vi "Heartbeat State Manager.vi"(8 "Error In":errorcluster, 9 "Heartbeat state manager Input VI names":T6, 11 "HB Command Event IN":refnum<user-event>) -> (0 "Error Out":errorcluster, 1 "Error conditions Cluster":T4, 2 "Master-Slave messaging Flags":T5={"Instruction available"=TRUE, "Slave action completed"=TRUE, "Slave Ready?"=FALSE}, 3 "Heartbeat information cluster":T1, 4 "Slave Completions Received":i32, 5 "Master Instructions Issued":i32)   [LabVIEW 2012]
doc: "SciScan 1.2 160622\nThis VI MUST be used in all VIs which make use of heartbeats for synchronisation with a client or slave"
uses:
  Heartbeat state manager Input VI names.ctl
  Master Slave messaging Flags.ctl
  Custom Controls and Typedefs/HB_Error Conditions Cluster.ctl
  Custom Controls and Typedefs/Heartbeat information cluster.ctl
  Custom Controls and Typedefs/Heartbeat Event Source.ctl
  Custom Controls/Heartbeat_States.ctl
  Custom Controls and Typedefs/HB Actionable Event.ctl
  Broken Chain FGV Command.ctl
  CommonResource VIs/Timing/Timer Commands.ctl
  Custom Controls and Typedefs/HFG Commands.ctl
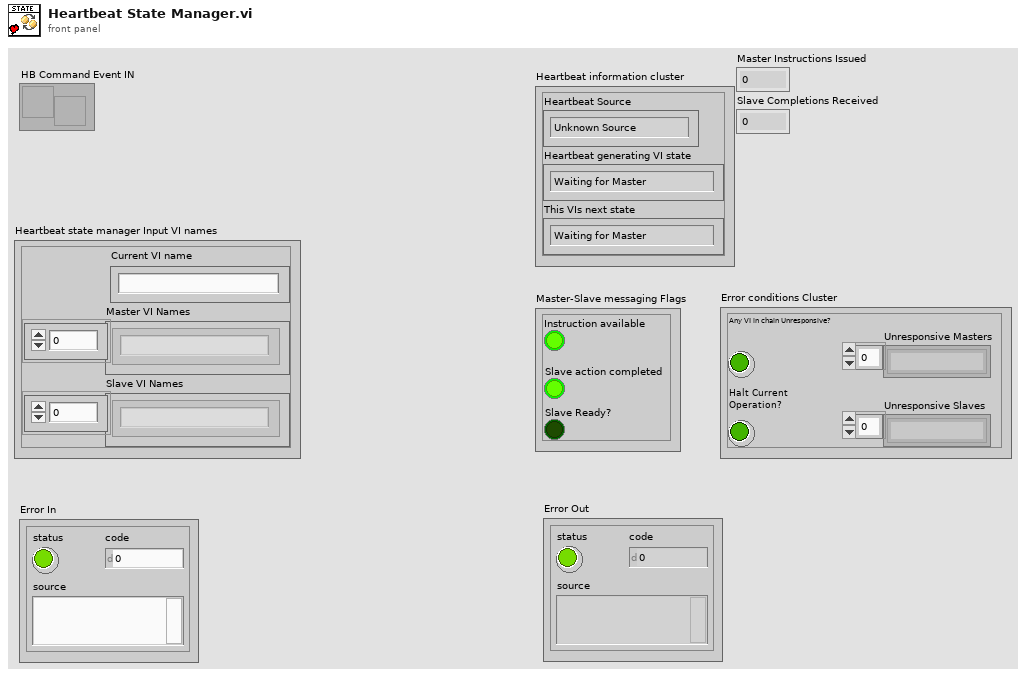
[diagram p1: front panel]
types:
  T1 = typedef "Heartbeat information cluster.ctl" = cluster{"Heartbeat Source":T2, "Heartbeat generating VI state":T3, "This VIs next state":T3}
  T2 = typedef "Heartbeat Event Source.ctl" = enum16{"Unknown Source", "Timeout", "This VI", "Master", "Slave"}
  T3 = typedef "Heartbeat_States.ctl" = enum16{"Waiting for Master", "Instruction Issued", "Waiting for Slave Completion", "Completed", "Cancelled", "Failed", "Broken Link"}
  T4 = typedef "HB_Error Conditions Cluster.ctl" = cluster{"Any VI in chain Unresponsive?":bool, "Halt Current Operation?":bool, "Unresponsive Masters":string[], "Unresponsive Slaves":string[]}
  T5 = typedef "Master Slave messaging Flags.ctl" = cluster{"Instruction available":bool, "Slave action completed":bool, "Slave Ready?":bool}
  T6 = typedef "Heartbeat state manager Input VI names.ctl" = cluster{"Current VI name":string, "Master VI Names":string[], "Slave VI Names":string[]}
  T7 = typedef "Broken Chain FGV Command.ctl" = enum16{"Initialize", "Update VI status", "Get All VI status"}
  T8 = cluster{"Master VI Names":string[], "Slave VI Names":string[]}
  T9 = typedef "HFG Commands.ctl" = enum16{"Set", "Get", "Initialize"}
  T10 = typedef "Timer Commands.ctl" = enum16{"Clear All", "Start", "Pause", "Check Time"}
  T11 = typedef "HB Actionable Event.ctl" = enum16{"Master instruction event", "Slave ready event", "Slave unavailable event", "Cancelled or Failed event", "Slave action complete event", "QUIT", "Broken Link", "Recovered from Broken Link"}
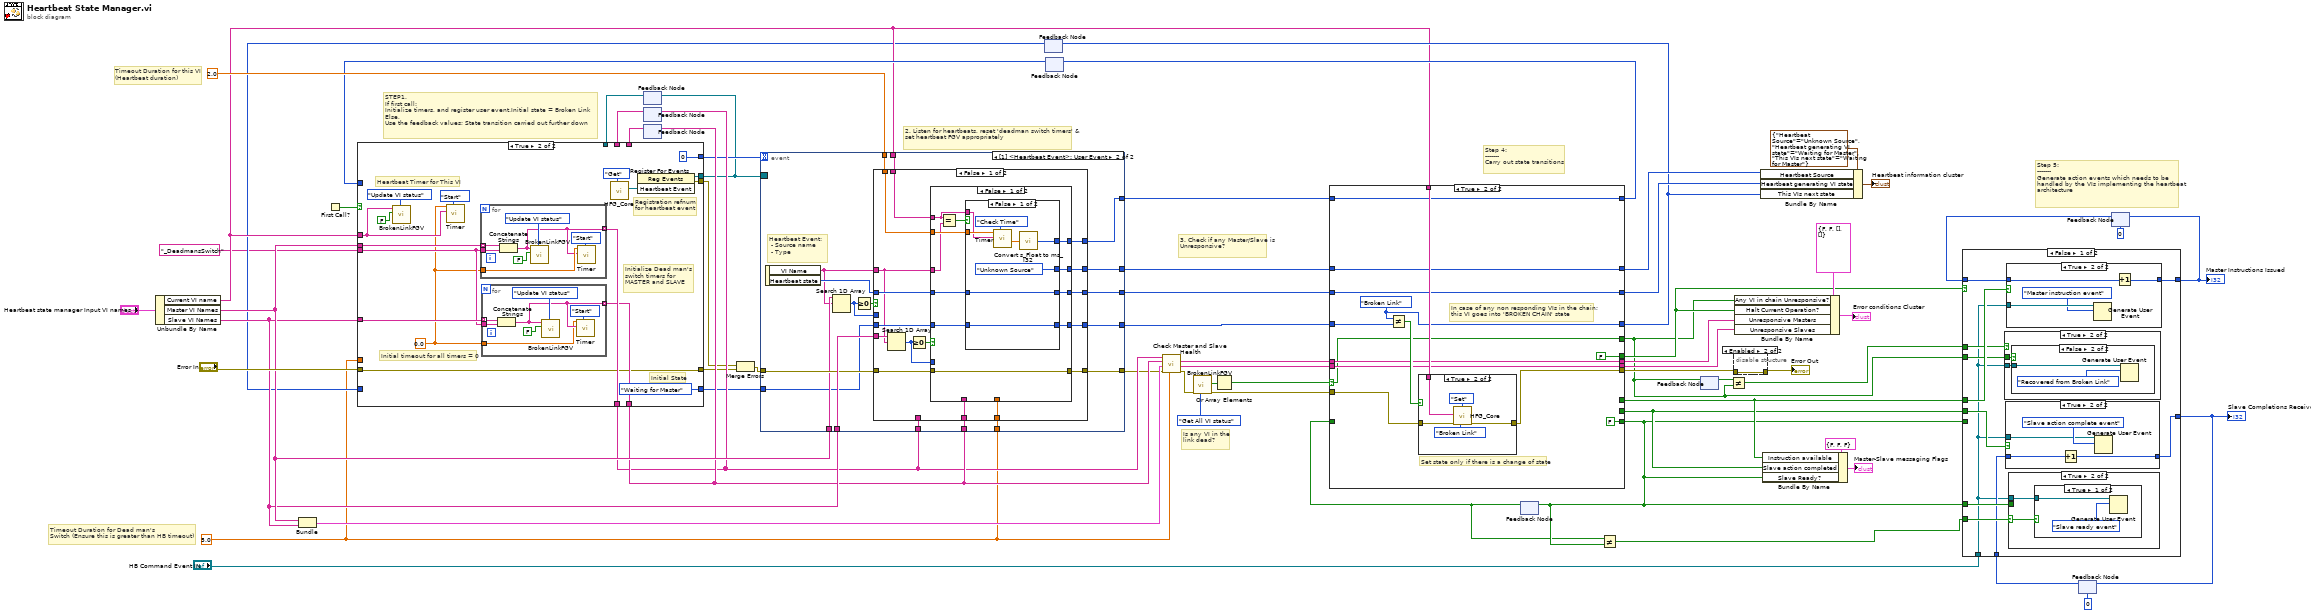
[diagram p0: block diagram]
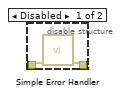
[diagram p2: hidden frame]
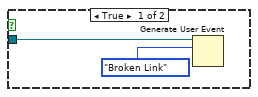
[diagram p4: hidden frame]
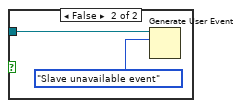
[diagram p7: hidden frame]
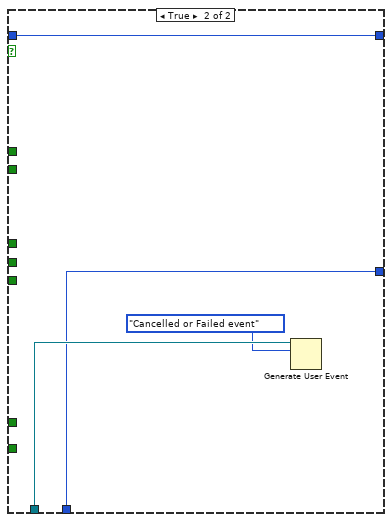
[diagram p9: hidden frame]
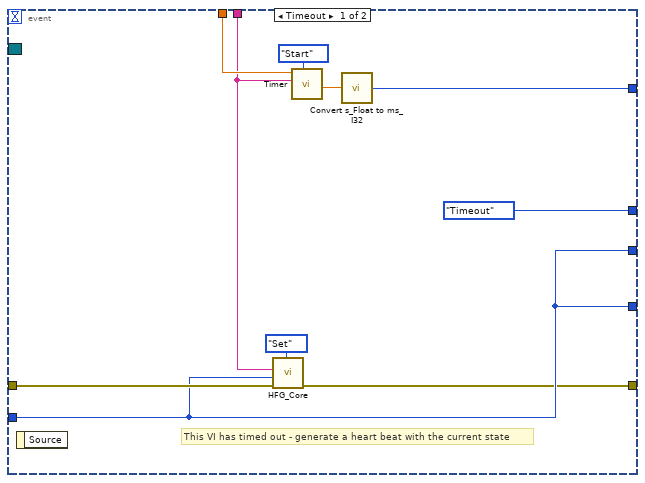
[diagram p10: hidden frame]
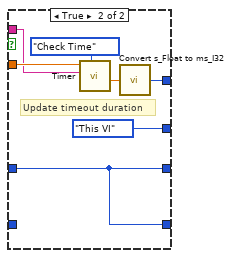
[diagram p11: hidden frame]
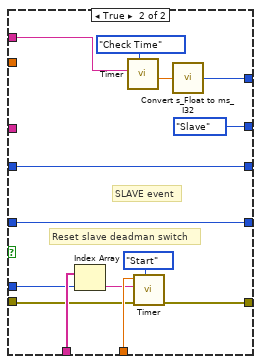
[diagram p12: hidden frame]
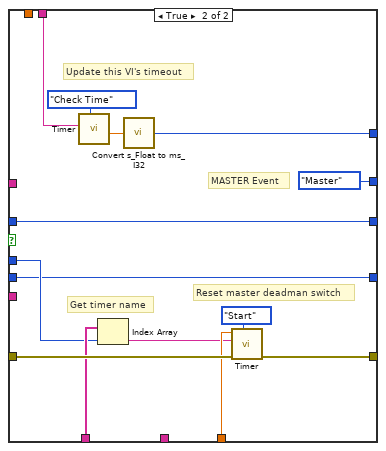
[diagram p13: hidden frame]
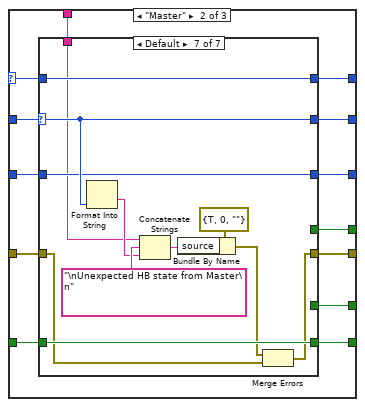
[diagram p16: hidden frame]
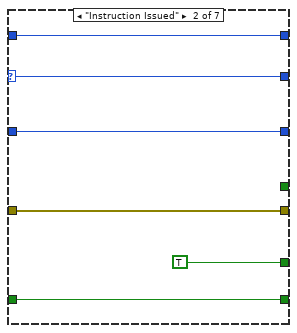
[diagram p18: hidden frame]
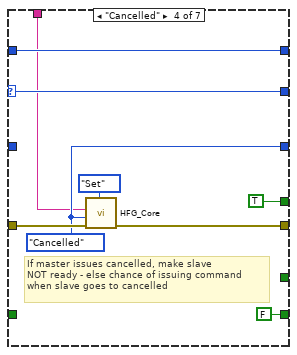
[diagram p20: hidden frame]
diagram:
  w27 = 5.0 ("Response time for Master/Slave")
  # "Timeout Duration for Dead man's\nSwitch (Ensure this is greater than HB timeout)"
  # "Step 5:\n-------\nGenerate action events which needs to be handled by the VIs implementing the heartbeat architecture"
  # "Is any VI in the link dead?"
  # "2. Listen for heartbeats, reset 'deadman switch timers' & set heartbeat FGV appropriately"
  # "Timeout Duration for this VI\n(Heartbeat duration)"
  # "Step 4:\n-------\nCarry out state transitions"
  # "3. Check if any Master/Slave is Unresponsive?"
  # "STEP1. \nIf first call:\nInitialize timers, and register user event.Initial state = Broken Link\nElse,\nUse the feedback values; State transition carried out further down"
  n1 = Unbundle By Name("Heartbeat state manager Input VI names") -> ("Current VI name"=w46:string, "Master VI Names"=w45:string[], "Slave VI Names"=w44:string[])
  n2 = Bundle("Master VI Names"=w45, "Slave VI Names"=w44) -> (w60:T8)  [unwired: 1 in]
  n3 = First Call?() -> (First Call?: T/F=w64:bool)
  n4 = feedback #1() -> (w33:refnum<event-registration>)  [unwired: 1 in]
  n5 = feedback #2() -> (w63:string[])  [unwired: 1 in]
  n6 = feedback #3() -> (w62:string[])  [unwired: 1 in]
  n7 = feedback #4() -> (w37:T3)  [unwired: 1 in]
  n8 = feedback #5() -> (w47:i32)  [unwired: 1 in]
  n9 = case shown="True" w64 {
    tunnel: w46 -> [_ w80]
    tunnel: w45 -> [_ w88]
    tunnel: w44 -> [_ w87]
    tunnel: [w71 w86] -> w42
    tunnel: [w70 w85] -> w43
    tunnel: w63 -> [w71 _]
    tunnel: w62 -> [w70 _]
    tunnel: [w69 w84] -> w2
    tunnel: "Error In" -> [w69 w84]
    tunnel: w27 -> [_ _]
    tunnel: [w68 0] -> w35
    tunnel: w47 -> [w68 _]
    tunnel: w37 -> [w67 _]
    tunnel: [w67 Heartbeat_States."Waiting for Master" ("x")] -> w36
    tunnel: [w66 w75] -> w34
    tunnel: w33 -> [w66 _]
    tunnel: "_DeadmansSwitch" ("Current VI name") -> [_ w74]
    tunnel: [_ w72] -> w1
    frame False {
    }
    frame True {
      w73 = 0.0 ("Response time for Master/Slave")
      # "Registration refnum\nfor heartbeat event"
      # "Initial State"
      # "Initialize Dead man's switch timers for MASTER and SLAVE"
      # "Heartbeat Timer for This VI"
      # "Initial timeout for all timers = 0"
      n10 = call "BrokenLinkFGV.vi"("Broken Chain FGV Action"=Broken_Chain_FGV_Command."Update VI status", "Broken?"=FALSE, "String"=w80) -> ()  [unwired: 6 in, 3 out]
      n11 = call "Timer.vi"("Timer Command"=Timer_Commands."Start", "VI name (Optional)"=w80, "Set Time IN (s)"=w73) -> ()  [unwired: 3 in, 6 out]
      n12 = for {
        tunnel: w88 -> [w100] mode=indexing
        tunnel: [w96] -> w86 mode=indexing
        tunnel: w74 -> [w99]
        tunnel: w73 -> [w97]
        n13 = Concatenate Strings(w100, w99) -> (w96:string)
        n14 = call "BrokenLinkFGV.vi"("Broken Chain FGV Action"=Broken_Chain_FGV_Command."Update VI status", "Broken?"=FALSE, "String"=w96) -> ()  [unwired: 6 in, 3 out]
        n15 = call "Timer.vi"("Timer Command"=Timer_Commands."Start", "VI name (Optional)"=w96, "Set Time IN (s)"=w97) -> ()  [unwired: 3 in, 6 out]
      }
      n16 = for {
        tunnel: w87 -> [w93] mode=indexing
        tunnel: [w90] -> w85 mode=indexing
        tunnel: w74 -> [w92]
        tunnel: w73 -> [w89]
        n17 = Concatenate Strings(w93, w92) -> (w90:string)
        n18 = call "BrokenLinkFGV.vi"("Broken Chain FGV Action"=Broken_Chain_FGV_Command."Update VI status", "Broken?"=FALSE, "String"=w90) -> ()  [unwired: 6 in, 3 out]
        n19 = call "Timer.vi"("Timer Command"=Timer_Commands."Start", "VI name (Optional)"=w90, "Set Time IN (s)"=w89) -> ()  [unwired: 3 in, 6 out]
      }
      n20 = call "HFG_Core.vi"("HFG Commands"=HFG_Commands."Get") -> ("Heartbeat Event"=w77:refnum<user-event>)  [unwired: 7 in, 3 out]
      n21 = register-events(w77) -> (reference out=w75:refnum<event-registration>, error out=w72:errorcluster)  [unwired: 2 in]
    }
  }
  n22 = feedback-in #1(w34) -> ()
  n23 = feedback-in #2(w42) -> ()
  n24 = feedback-in #3(w43) -> ()
  n25 = Merge Errors(w1, w2) -> (w3:errorcluster)
  n26 = event shown="[1] <Heartbeat Event>: User Event" {
    selector: w34 -> [_ _]
    dyn-events: _ -> [_ _]
    timeout: w35 -> [_ _]
    tunnel: w36 -> [w105 w120]
    tunnel: [w105 w114] -> w24
    tunnel: 2.0 ("Response time for Master/Slave") -> [w111 w129]
    tunnel: [w106 w128] -> w38
    tunnel: [w105 w117] -> w40
    tunnel: w46 -> [w103 w130]
    tunnel: w3 -> [w109 w123]
    tunnel: [w104 w115] -> w41
    tunnel: [Heartbeat_Event_Source."Timeout" ("Heartbeat Event Types") w127] -> w39
    tunnel: w45 -> [_ w122]
    tunnel: w44 -> [_ w126]
    tunnel: w43 -> [_ w125]
    tunnel: w27 -> [_ w124]
    tunnel: w42 -> [_ w116]
    event Timeout {
      # "This VI has timed out - generate a heart beat with the current state"
      n27 = event-data() -> ()  [unwired: 1 in, 1 out]
      n28 = call "HFG_Core.vi"("HFG Commands"=HFG_Commands."Set", "Error In"=w109, "Heartbeat state IN"=w105, "VI Name (Calling VIs name by default)"=w103) -> ("Error Out"=w104:errorcluster)  [unwired: 4 in, 3 out]
      n29 = call "Timer.vi"("Timer Command"=Timer_Commands."Start", "VI name (Optional)"=w103, "Set Time IN (s)"=w111) -> ("Remaining Time (s)"=w107:dbl)  [unwired: 3 in, 5 out]
      n30 = call "Convert s_Float to ms_I32.vi"("Seconds IN (Float)"=w107) -> ("milliseconds OUT (I32)"=w106:i32)
    }
    event User Event {
      # "Heartbeat Event: \n - Source name\n - Type"
      n31 = event-data() -> ("VI Name"=w113:string, "Heartbeat state"=w118:T3)  [unwired: 1 in]
      n32 = Search 1D Array(1D array=w122, element=w113) -> (index of element=w119:i32)  [unwired: 1 in]
      n33 = Greater Or Equal To 0?(x=w119) -> (x >= 0?=w121:bool)
      n34 = case shown="False" w121 {
        tunnel: w130 -> [w146 w198]
        tunnel: w129 -> [w145 _]
        tunnel: [w144 w197] -> w128
        tunnel: [w143 Heartbeat_Event_Source."Master" ("Heartbeat Event Types")] -> w127
        tunnel: w113 -> [w131 _]
        tunnel: w126 -> [w142 _]
        tunnel: w125 -> [w140 _]
        tunnel: w124 -> [w139 w191]
        tunnel: w123 -> [w137 w194]
        tunnel: w120 -> [w134 w189]
        tunnel: w119 -> [_ w192]
        tunnel: w118 -> [w136 w195]
        tunnel: [w135 w195] -> w117
        tunnel: w116 -> [_ w193]
        tunnel: [w133 w190] -> w115
        tunnel: [w132 w189] -> w114
        frame False {
          n35 = Search 1D Array(1D array=w142, element=w131) -> (index of element=w138:i32)  [unwired: 1 in]
          n36 = Greater Or Equal To 0?(x=w138) -> (x >= 0?=w141:bool)
          n37 = case shown="False" w141 {
            tunnel: w146 -> [w147 w178]
            tunnel: w145 -> [w156 _]
            tunnel: [w155 w180] -> w144
            tunnel: [w154 Heartbeat_Event_Source."Slave" ("Heartbeat Event Types")] -> w143
            tunnel: w131 -> [w153 _]
            tunnel: w140 -> [_ w185]
            tunnel: w139 -> [_ w184]
            tunnel: w138 -> [_ w183]
            tunnel: w137 -> [w152 w179]
            tunnel: w136 -> [w151 w176]
            tunnel: [w149 w176] -> w135
            tunnel: w134 -> [w148 w175]
            tunnel: [w152 w177] -> w133
            tunnel: [w150 w175] -> w132
            frame False {
              n38 = Equal?(x=w147, y=w153) -> (x = y?=w157:bool)
              n39 = case shown="False" w157 {
                tunnel: w156 -> [w164 w171]
                tunnel: [w162 w169] -> w155
                tunnel: [Heartbeat_Event_Source."Unknown Source" ("Heartbeat Event Types") Heartbeat_Event_Source."This VI" ("Heartbeat Event Types")] -> w154
                tunnel: w151 -> [w160 w167]
                tunnel: [w159 w167] -> w150
                tunnel: [w160 w167] -> w149
                tunnel: w148 -> [w159 _]
                tunnel: w147 -> [w158 w166]
                frame False {
                  n40 = call "Timer.vi"("Timer Command"=Timer_Commands."Check Time", "VI name (Optional)"=w158, "Set Time IN (s)"=w164) -> ("Remaining Time (s)"=w163:dbl)  [unwired: 3 in, 5 out]
                  n41 = call "Convert s_Float to ms_I32.vi"("Seconds IN (Float)"=w163) -> ("milliseconds OUT (I32)"=w162:i32)
                }
                frame True {
                  # "Update timeout duration"
                  n42 = call "Timer.vi"("Timer Command"=Timer_Commands."Check Time", "VI name (Optional)"=w166, "Set Time IN (s)"=w171) -> ("Remaining Time (s)"=w170:dbl)  [unwired: 3 in, 5 out]
                  n43 = call "Convert s_Float to ms_I32.vi"("Seconds IN (Float)"=w170) -> ("milliseconds OUT (I32)"=w169:i32)
                }
              }
            }
            frame True {
              # "Reset slave deadman switch"
              # "SLAVE event"
              n44 = Index Array(array=w185, index=w183) -> (element=w173:string)
              n45 = call "Timer.vi"("Timer Command"=Timer_Commands."Check Time", "VI name (Optional)"=w178) -> ("Remaining Time (s)"=w181:dbl)  [unwired: 4 in, 5 out]
              n46 = call "Timer.vi"("Timer Command"=Timer_Commands."Start", "Error In"=w179, "VI name (Optional)"=w173, "Set Time IN (s)"=w184) -> ("Error Out"=w177:errorcluster)  [unwired: 2 in, 5 out]
              n47 = call "Convert s_Float to ms_I32.vi"("Seconds IN (Float)"=w181) -> ("milliseconds OUT (I32)"=w180:i32)
            }
          }
        }
        frame True {
          # "Get timer name"
          # "Update this VI's timeout"
          # "Reset master deadman switch"
          # "MASTER Event"
          n48 = call "Timer.vi"("Timer Command"=Timer_Commands."Check Time", "VI name (Optional)"=w198) -> ("Remaining Time (s)"=w199:dbl)  [unwired: 4 in, 5 out]
          n49 = Index Array(array=w193, index=w192) -> (element=w187:string)
          n50 = call "Convert s_Float to ms_I32.vi"("Seconds IN (Float)"=w199) -> ("milliseconds OUT (I32)"=w197:i32)
          n51 = call "Timer.vi"("Timer Command"=Timer_Commands."Start", "Error In"=w194, "VI name (Optional)"=w187, "Set Time IN (s)"=w191) -> ("Error Out"=w190:errorcluster)  [unwired: 2 in, 5 out]
        }
      }
    }
  }
  n52 = call "Check Master and Slave Health.vi"("Timeout duration"=w27, "Error In"=w41, "Master and Slave VI names"=w60, "Slave timer names array"=w43, "Master timer names array"=w42) -> ("Error Out"=w30:errorcluster, "Unresponsive Slaves"=w7:string[], "Unresponsive Masters"=w8:string[])  [unwired: 3 in, 1 out]
  n53 = call "BrokenLinkFGV.vi"("Broken Chain FGV Action"=Broken_Chain_FGV_Command."Get All VI status", "Error In"=w30) -> ("Error Out"=w28:errorcluster, "VI broken? array"=w32:bool[])  [unwired: 7 in, 1 out]
  n54 = Or Array Elements(Boolean array=w32) -> (logical OR=w29:bool)
  n55 = feedback #6() -> (w13:bool)  [unwired: 1 in]
  n56 = case shown="True" w29 {
    selector: w29 -> [_ w528]
    tunnel: w28 -> [w213 w539]
    tunnel: w24 -> [w215 w541]
    tunnel: w40 -> [w210 w536]
    tunnel: w39 -> [w208 w535]
    tunnel: [w202 FALSE ("Halt Current Operation")] -> w16
    tunnel: w46 -> [w212 w538]
    tunnel: [w214 w537] -> w50
    tunnel: [w209 w536] -> w52
    tunnel: [w207 w535] -> w51
    tunnel: [_ w528] -> w4
    tunnel: w8 -> [_ w534]
    tunnel: w7 -> [_ w533]
    tunnel: [_ w534] -> w55
    tunnel: [_ w533] -> w54
    tunnel: [w211 w531] -> w26
    tunnel: [w206 _] -> w21
    tunnel: [w205 _] -> w15
    tunnel: [w204 FALSE] -> w14
    tunnel: w13 -> [w203 _]
    tunnel: w38 -> [w201 w529]
    tunnel: [w201 w529] -> w48
    frame False {
      n57 = case shown="\"Waiting for Master\"" w215 {
        selector: w215 -> [w224 _ w397 _ _]
        tunnel: [w225 w350 w398 w515 w526] -> w214
        tunnel: w213 -> [w220 w345 w393 w517 w521]
        tunnel: w212 -> [w219 w351 w392 w516 w527]
        tunnel: [w221 w344 w394 w514 w525] -> w211
        tunnel: [w223 w347 w396 w519 w523] -> w209
        tunnel: w210 -> [w227 w348 w400 w519 w523]
        tunnel: [w222 w346 w395 w520 w524] -> w207
        tunnel: w208 -> [w228 w349 w401 w520 w524]
        tunnel: [w226 _ w399 _ _] -> w206
        tunnel: [_ _ w391 _ _] -> w205
        tunnel: [w218 w342 w389 _ _] -> w204
        tunnel: w203 -> [w217 w343 w388 _ _]
        tunnel: [w216 w341 w390 _ _] -> w202
        frame "Waiting for Master" {
          n58 = case shown="\"Slave\"" w228 {
            selector: w228 -> [w233 w240 w299]
            tunnel: w227 -> [w232 w246 w304]
            tunnel: [_ w245 _] -> w226
            tunnel: [w231 w244 w303] -> w225
            tunnel: w224 -> [w231 w243 w302]
            tunnel: [w232 w242 w301] -> w223
            tunnel: [w233 w241 w300] -> w222
            tunnel: [w230 w239 w298] -> w221
            tunnel: w220 -> [w230 w238 w297]
            tunnel: w219 -> [_ w237 w296]
            tunnel: [w229 w235 w295] -> w218
            tunnel: w217 -> [w229 w236 w294]
            tunnel: [_ w234 _] -> w216
            frame Default {
            }
            frame "Master" {
              n59 = case shown="Default" w246 {
                selector: w246 -> [w250 w254 w261 w270 w275 w280 w284]
                tunnel: [_ TRUE _ _ _ _ _] -> w245
                tunnel: [w249 w256 w260 w266 w274 w279 w283] -> w244
                tunnel: w243 -> [w249 w256 w260 _ w274 w279 w283]
                tunnel: [w250 w254 w261 w270 w275 w280 w284] -> w242
                tunnel: [w251 w253 w262 w271 w276 w281 w285] -> w241
                tunnel: w240 -> [w251 w253 w262 w271 w276 w281 w285]
                tunnel: [w248 w255 w259 w267 w273 w278 w286] -> w239
                tunnel: w238 -> [w248 w255 w259 w268 w273 w278 w287]
                tunnel: w237 -> [_ _ _ w265 _ _ w282]
                tunnel: [w247 w252 w258 FALSE w272 FALSE w293] -> w235
                tunnel: w236 -> [w247 w252 w258 _ w272 _ w293]
                tunnel: [_ _ _ TRUE _ _ _] -> w234
                frame "Waiting for Master" {
                  # "New case added"
                }
                frame "Instruction Issued" {
                }
                frame "Waiting for Slave Completion" {
                  # "Master might issue a command and go\nto 'waiting for slave completion'\n- This VI has a lag to get the \n'instruction issued' command"
                  # "New case added"
                }
                frame "Cancelled" {
                  w266 = Heartbeat_States."Cancelled" ("This VIs previous Heartbeat state")
                  # "If master issues cancelled, make slave\nNOT ready - else chance of issuing command\nwhen slave goes to cancelled"
                  n60 = call "HFG_Core.vi"("HFG Commands"=HFG_Commands."Set", "Error In"=w268, "Heartbeat state IN"=w266, "VI Name (Calling VIs name by default)"=w265) -> ("Error Out"=w267:errorcluster)  [unwired: 4 in, 3 out]
                }
                frame "Completed" {
                  # "Master might issue a 'Completed' \n- after This VI issues a 'Completed', and \nalready reached 'Waiting for Master' \ncommand.\n- This is due to lag"
                  # "New case added"
                }
                frame "Broken Link" {
                  # "New case added"
                }
                frame Default {
                  n61 = Format Into String(w284) -> (resulting string=w289:string)  [unwired: 3 in, 1 out]
                  n62 = Concatenate Strings(w282, "\nUnexpected HB state from Master\n" ("source"), w289) -> (w291:string)
                  n63 = Bundle By Name(cluster=errorcluster {"status"=TRUE, "code"=0, "source"=""} ("error in (no error)"), "source"=w291) -> (w288:errorcluster)
                  n64 = Merge Errors(w288, w287) -> (w286:errorcluster)
                }
              }
            }
            frame "Slave" {
              n65 = case shown="\"Cancelled\"" w304 {
                selector: w304 -> [w305 w311 w315 w319 w323 w327 w331]
                tunnel: [w307 w312 w316 w320 w324 w328 w336] -> w303
                tunnel: w302 -> [w307 w312 w316 w320 w324 w328 w336]
                tunnel: [w305 w311 w315 w319 w323 w327 w331] -> w301
                tunnel: [w306 w310 w314 w318 w322 w326 w340] -> w300
                tunnel: w299 -> [w306 w310 w314 w318 w322 w326 w340]
                tunnel: [w308 w313 w317 w321 w325 w329 w338] -> w298
                tunnel: w297 -> [w308 w313 w317 w321 w325 w329 w339]
                tunnel: w296 -> [_ _ _ _ _ _ w330]
                tunnel: [TRUE _ _ _ _ _ _] -> w295
                tunnel: w294 -> [_ _ _ _ _ _ _]
                frame "Waiting for Master" {
                }
                frame "Instruction Issued" {
                  # "New case - else error\nThis one is for ' lag in slave receiving cancelled'\nOnce master issues a cancel and goes into\n'Wait for master' state, the slave might do an\n'instruction issued' for a task in progress"
                }
                frame "Waiting for Slave Completion" {
                  # "New case - else error\nThis one is for ' lag in slave receiving cancelled'\nOnce master issues a cancel and goes into\n'Wait for master' state, the slave might have done\n'instruction issued'  and  move to 'waiting for slave \ncompletion'"
                }
                frame "Cancelled" {
                  # "New case - else error\nOnce master issues a cancel and goes into\n'Wait for master' state, the slave would issue its\nown cancelled as it travels downstream"
                }
                frame "Completed" {
                  # "New case - else error\nThis one is for 'late finishers'\nOnce master issues a cancel and goes into\n'Wait for master' state, the slave might issue a \ncompleted for a command previously completed"
                }
                frame "Broken Link" {
                }
                frame Default {
                  n66 = Format Into String(w331) -> (resulting string=w333:string)  [unwired: 3 in, 1 out]
                  n67 = Concatenate Strings(w330, "\nUnexpected HB state from slave\n" ("source"), w333) -> (w335:string)
                  n68 = Bundle By Name(cluster=errorcluster {"status"=TRUE, "code"=0, "source"=""} ("error in (no error)"), "source"=w335) -> (w332:errorcluster)
                  n69 = Merge Errors(w332, w339) -> (w338:errorcluster)
                }
              }
            }
          }
        }
        frame "Instruction Issued" {
          n70 = case shown="\"Master\"" w349 {
            selector: w349 -> [w355 w365]
            tunnel: w351 -> [w357 w370]
            tunnel: [w358 w369] -> w350
            tunnel: w348 -> [w356 w368]
            tunnel: [w356 w367] -> w347
            tunnel: [w355 w366] -> w346
            tunnel: w345 -> [w354 w364]
            tunnel: [w353 w363] -> w344
            tunnel: w343 -> [w352 w362]
            tunnel: [w352 w361] -> w342
            tunnel: [_ w360] -> w341
            frame Default {
              w358 = Heartbeat_States."Waiting for Slave Completion" ("VI State")
              # "If not special case of\ncancellation by master,\ngo to 'Wait for Slave Completion'"
              n71 = call "HFG_Core.vi"("HFG Commands"=HFG_Commands."Set", "Error In"=w354, "Heartbeat state IN"=w358, "VI Name (Calling VIs name by default)"=w357) -> ("Error Out"=w353:errorcluster)  [unwired: 4 in, 3 out]
            }
            frame "Master" {
              n72 = case shown="Default" w368 {
                selector: w368 -> [w375 w384]
                tunnel: w370 -> [w376 w386]
                tunnel: [w377 w385] -> w369
                tunnel: [w375 w384] -> w367
                tunnel: [w374 w383] -> w366
                tunnel: w365 -> [w374 w383]
                tunnel: w364 -> [w373 w382]
                tunnel: [w372 w381] -> w363
                tunnel: w362 -> [w371 _]
                tunnel: [w371 FALSE] -> w361
                tunnel: [_ TRUE] -> w360
                frame Default {
                  w377 = Heartbeat_States."Waiting for Slave Completion" ("VI State")
                  # "If not special case of\ncancellation by master,\ngo to 'Wait for Slave Completion'"
                  n73 = call "HFG_Core.vi"("HFG Commands"=HFG_Commands."Set", "Error In"=w373, "Heartbeat state IN"=w377, "VI Name (Calling VIs name by default)"=w376) -> ("Error Out"=w372:errorcluster)  [unwired: 4 in, 3 out]
                }
                frame "Cancelled" {
                  w385 = Heartbeat_States."Cancelled" ("VI State")
                  # "If master issues cancelled, make slave\nNOT ready - else chance of issuing command when slave goes to cancelled"
                  # "'Cancelled 'by Master.\nChange state to 'Cancelled'"
                  n74 = call "HFG_Core.vi"("HFG Commands"=HFG_Commands."Set", "Error In"=w382, "Heartbeat state IN"=w385, "VI Name (Calling VIs name by default)"=w386) -> ("Error Out"=w381:errorcluster)  [unwired: 4 in, 3 out]
                }
              }
            }
          }
        }
        frame "Waiting for Slave Completion" {
          n75 = case shown="\"Slave\"" w401 {
            selector: w401 -> [w408 w457 w513]
            tunnel: w400 -> [w414 w462 w512]
            tunnel: [w413 _ _] -> w399
            tunnel: [w412 w461 w511] -> w398
            tunnel: w397 -> [w411 w460 w511]
            tunnel: [w410 w459 w512] -> w396
            tunnel: [w409 w458 w513] -> w395
            tunnel: [w407 w456 w510] -> w394
            tunnel: w393 -> [w406 w455 w510]
            tunnel: w392 -> [w405 w454 _]
            tunnel: [_ w453 _] -> w391
            tunnel: [w404 w452 _] -> w390
            tunnel: [w402 w451 w509] -> w389
            tunnel: w388 -> [w403 w450 w509]
            frame "Master" {
              n76 = case shown="Default" w414 {
                selector: w414 -> [w423 w428 w433 w437 w440]
                tunnel: [FALSE _ _ _ _] -> w413
                tunnel: [w419 w426 w430 w435 w443] -> w412
                tunnel: w411 -> [_ w426 w430 w435 w443]
                tunnel: [w423 w428 w433 w437 w440] -> w410
                tunnel: [w424 w429 w434 w438 w449] -> w409
                tunnel: w408 -> [w424 w429 w434 w438 w449]
                tunnel: [w420 w427 w431 w436 w447] -> w407
                tunnel: w406 -> [w421 w427 w431 w436 w448]
                tunnel: w405 -> [w418 _ _ _ w439]
                tunnel: [TRUE _ FALSE _ _] -> w404
                tunnel: w403 -> [_ w425 _ _ _]
                tunnel: [FALSE w425 _ _ _] -> w402
                frame "Cancelled" {
                  w419 = Heartbeat_States."Cancelled" ("This VIs previous Heartbeat state")
                  # "If master issues cancelled, make slave\nNOT ready - else chance of issuing command when slave goes to cancelled"
                  n77 = call "HFG_Core.vi"("HFG Commands"=HFG_Commands."Set", "Error In"=w421, "Heartbeat state IN"=w419, "VI Name (Calling VIs name by default)"=w418) -> ("Error Out"=w420:errorcluster)  [unwired: 4 in, 3 out]
                }
                frame "Waiting for Slave Completion" {
                  # "New case - else error being issued"
                }
                frame "Waiting for Master" {
                  # "Scenario where master 'Canceled' and has\ngone to 'Waiting for Master'.\n\nThe 'Cancelled' has not reached This VI\ndue to lag"
                  # "New case - else error being issued"
                }
                frame "Broken Link" {
                  # "New case - else error being issued"
                }
                frame Default {
                  n78 = Format Into String(w440) -> (resulting string=w442:string)  [unwired: 3 in, 1 out]
                  n79 = Concatenate Strings(w439, "\nUnexpected HB state from Master\n" ("source"), w442) -> (w445:string)
                  n80 = Bundle By Name(cluster=errorcluster {"status"=TRUE, "code"=0, "source"=""} ("error in (no error)"), "source"=w445) -> (w441:errorcluster)
                  n81 = Merge Errors(w441, w448) -> (w447:errorcluster)
                }
              }
            }
            frame "Slave" {
              n82 = case shown="\"Completed\"" w462 {
                selector: w462 -> [w464 w468 w474 w483 w487 w491 w495 w503]
                tunnel: [w466 w470 w476 w479 w486 w493 w497 w507] -> w461
                tunnel: w460 -> [w466 w470 w476 _ w486 w493 w497 w507]
                tunnel: [w464 w468 w474 w483 w487 w491 w495 w503] -> w459
                tunnel: [w463 w467 w473 w484 w488 w490 w494 w508] -> w458
                tunnel: w457 -> [w463 w467 w473 w484 w488 w490 w494 w508]
                tunnel: [w465 w469 w475 w480 w485 w492 w496 w505] -> w456
                tunnel: w455 -> [w465 w469 w475 w481 w485 w492 w496 w506]
                tunnel: w454 -> [_ _ _ w478 _ _ _ w501]
                tunnel: [_ _ TRUE _ _ _ _ _] -> w453
                tunnel: [_ _ _ TRUE _ _ _ _] -> w452
                tunnel: [_ _ w471 _ TRUE _ _ _] -> w451
                tunnel: w450 -> [_ _ w471 _ _ _ _ _]
                frame "Waiting for Slave Completion" {
                }
                frame "Instruction Issued" {
                  # "Slave has issued instruction further\ndown the chain"
                }
                frame "Completed" {
                }
                frame "Failed" {
                  w479 = Heartbeat_States."Failed" ("This VIs previous Heartbeat state")
                  # "If slave fails, set state of current VI to FAIL\nand halt current operation"
                  n83 = call "HFG_Core.vi"("HFG Commands"=HFG_Commands."Set", "Error In"=w481, "Heartbeat state IN"=w479, "VI Name (Calling VIs name by default)"=w478) -> ("Error Out"=w480:errorcluster)  [unwired: 4 in, 3 out]
                }
                frame "Waiting for Master" {
                }
                frame "Cancelled" {
                  # "New addition - else rare error while cancelling\nimmediately after an 'Instruction Issued'.\n\nBefore This VI can get to Cancelled state,\na slave could get into cancelled state"
                }
                frame "Broken Link" {
                }
                frame Default {
                  n84 = Format Into String(w503) -> (resulting string=w502:string)  [unwired: 3 in, 1 out]
                  n85 = Concatenate Strings(w501, "\nUnexpected HB state from slave\n" ("source"), w502) -> (w499:string)
                  n86 = Bundle By Name(cluster=errorcluster {"status"=TRUE, "code"=0, "source"=""} ("error in (no error)"), "source"=w499) -> (w498:errorcluster)
                  n87 = Merge Errors(w498, w506) -> (w505:errorcluster)
                }
              }
            }
            frame Default {
            }
          }
        }
        frame "Completed".."Failed" {
          w515 = Heartbeat_States."Waiting for Master" ("Heartbeat state IN")
          n88 = call "HFG_Core.vi"("HFG Commands"=HFG_Commands."Set", "Error In"=w517, "Heartbeat state IN"=w515, "VI Name (Calling VIs name by default)"=w516) -> ("Error Out"=w514:errorcluster)  [unwired: 4 in, 3 out]
        }
        frame "Broken Link" {
          w526 = Heartbeat_States."Waiting for Master" ("VI State")
          n89 = call "HFG_Core.vi"("HFG Commands"=HFG_Commands."Set", "Error In"=w521, "Heartbeat state IN"=w526, "VI Name (Calling VIs name by default)"=w527) -> ("Error Out"=w525:errorcluster)  [unwired: 4 in, 3 out]
        }
      }
    }
    frame True {
      w537 = Heartbeat_States."Broken Link" ("x")
      # "Set state only if there is a change of state"
      # "In case of any non responding VIs in the chain;\nthis VI goes into 'BROKEN CHAIN' state"
      n90 = Not Equal?(x=w537, y=w541) -> (x != y?=w540:bool)
      n91 = case shown="True" w540 {
        tunnel: w539 -> [w542 w545]
        tunnel: w538 -> [_ w544]
        tunnel: [w542 w543] -> w531
        frame False {
        }
        frame True {
          n92 = call "HFG_Core.vi"("HFG Commands"=HFG_Commands."Set", "Error In"=w545, "Heartbeat state IN"=Heartbeat_States."Broken Link" ("VI State"), "VI Name (Calling VIs name by default)"=w544) -> ("Error Out"=w543:errorcluster)  [unwired: 4 in, 3 out]
        }
      }
    }
  }
  n93 = feedback-in #4(w50) -> ()
  n94 = feedback-in #5(w48) -> ()
  n95 = feedback-in #6(w14) -> ()
  n96 = Not Equal?(x=w13, y=w14) -> (x != y?=w6:bool)
  n97 = feedback-in #7(w4) -> ()
  n98 = feedback #7() -> (w12:bool)  [unwired: 1 in]
  n99 = Not Equal?(x=w12, y=w4) -> (x != y?=w5:bool)
  n100 = disable-structure shown="Enabled" {
    disable-tunnel: w26 -> [w549 w550]
    disable-tunnel: [w548 w550] -> w25
    frame Disabled {
      n101 = call <vilib>:"Simple Error Handler.vi"("error in (no error)"=w549) -> ("error out"=w548:errorcluster)  [unwired: 4 in, 4 out]
    }
    frame Enabled {
    }
  }
  "Error Out" <- w25
  n102 = Bundle By Name(cluster=T4 {"Any VI in chain Unresponsive?"=FALSE, "Halt Current Operation?"=FALSE, "Unresponsive Masters"=[], "Unresponsive Slaves"=[]} ("Error conditions Cluster"), "Any VI in chain Unresponsive?"=w4, "Halt Current Operation?"=w16, "Unresponsive Masters"=w55, "Unresponsive Slaves"=w54) -> (→"Error conditions Cluster":T4)
  n103 = Bundle By Name(cluster=T1 {"Heartbeat Source"=enum."Unknown Source", "Heartbeat generating VI state"=enum."Waiting for Master", "This VIs next state"=enum."Waiting for Master"} ("Heartbeat information cluster"), "Heartbeat Source"=w51, "Heartbeat generating VI state"=w52, "This VIs next state"=w50) -> (→"Heartbeat information cluster":T1)
  n104 = Bundle By Name(cluster=T5 {"Instruction available"=FALSE, "Slave action completed"=FALSE, "Slave Ready?"=FALSE} ("Status Flags"), "Instruction available"=w21, "Slave action completed"=w15, "Slave Ready?"=w14) -> (→"Master-Slave messaging Flags":T5)
  n105 = feedback #8(0) -> (w11:i32)
  n106 = feedback #9(0) -> (w18:i32)
  n107 = case shown="False" w16 {
    tunnel: "HB Command Event IN" -> [w551 w587]
    tunnel: w21 -> [w561 _]
    tunnel: w15 -> [w556 _]
    tunnel: w14 -> [_ _]
    tunnel: w14 -> [w558 _]
    tunnel: [w560 w585] -> w20
    tunnel: w18 -> [w559 w585]
    tunnel: w6 -> [w557 _]
    tunnel: w11 -> [w555 w584]
    tunnel: [w554 w584] -> w10
    tunnel: w5 -> [w553 _]
    tunnel: w4 -> [w552 _]
    frame False {
      n108 = case shown="True" w553 {
        tunnel: w552 -> [_ w563]
        tunnel: w551 -> [_ w562]
        frame False {
        }
        frame True {
          n109 = case shown="False" w563 {
            tunnel: w562 -> [w565 w567]
            frame True {
              n110 = Generate User Event(user event=w565, event data cluster=HB_Actionable_Event."Broken Link" ("event data")) -> ()  [unwired: 1 in, 2 out]
            }
            frame False {
              n111 = Generate User Event(user event=w567, event data cluster=HB_Actionable_Event."Recovered from Broken Link" ("event data")) -> ()  [unwired: 1 in, 2 out]
            }
          }
        }
      }
      n112 = case shown="True" w556 {
        tunnel: w551 -> [_ w571]
        tunnel: w555 -> [w568 w570]
        tunnel: [w568 w569] -> w554
        frame False {
        }
        frame True {
          n113 = Increment(x=w570) -> (x+1=w569:i32)
          n114 = Generate User Event(user event=w571, event data cluster=HB_Actionable_Event."Slave action complete event" ("event data")) -> ()  [unwired: 1 in, 2 out]
        }
      }
      n115 = case shown="True" w561 {
        tunnel: w551 -> [_ w583]
        tunnel: [w579 w581] -> w560
        tunnel: w559 -> [w579 w580]
        frame False {
        }
        frame True {
          n116 = Generate User Event(user event=w583, event data cluster=HB_Actionable_Event."Master instruction event" ("event data")) -> ()  [unwired: 1 in, 2 out]
          n117 = Increment(x=w580) -> (x+1=w581:i32)
        }
      }
      n118 = case shown="True" w557 {
        selector: w557 -> [_ w573]
        tunnel: w551 -> [_ w574]
        tunnel: w558 -> [_ _]
        frame False {
        }
        frame True {
          n119 = case shown="True" w573 {
            tunnel: w574 -> [w576 w578]
            frame True {
              n120 = Generate User Event(user event=w576, event data cluster=HB_Actionable_Event."Slave ready event" ("element")) -> ()  [unwired: 1 in, 2 out]
            }
            frame False {
              n121 = Generate User Event(user event=w578, event data cluster=HB_Actionable_Event."Slave unavailable event" ("element")) -> ()  [unwired: 1 in, 2 out]
            }
          }
        }
      }
    }
    frame True {
      n122 = Generate User Event(user event=w587, event data cluster=HB_Actionable_Event."Cancelled or Failed event" ("event data")) -> ()  [unwired: 1 in, 2 out]
    }
  }
  "Master Instructions Issued" <- w20
  "Slave Completions Received" <- w10
  n123 = feedback-in #8(w10) -> ()
  n124 = feedback-in #9(w20) -> ()
